vi "Get_Indexes_Connect_Dots&Min_ID-1.vi"(4 "(X,Y...) Tracks col":dbl[](array[numeric]), 5 "ID-dot col":u16[](array[numeric]), 6 "multiplier (x4)":i32, 7 "dot status":i16, 8 "initial ID":u16, 9 "Current Dot \nindex":i32, 10 "Dot coord":cluster{"X":dbl, "Y":dbl, "dX":dbl, "dY":dbl}, 11 "N elem. in col":i32) -> (0 "minimal ID \nbetween them":u16, 1 "amount":i32, 2 "Indexex Connec\ndots":i32[](array[numeric]))   [LabVIEW 2013]
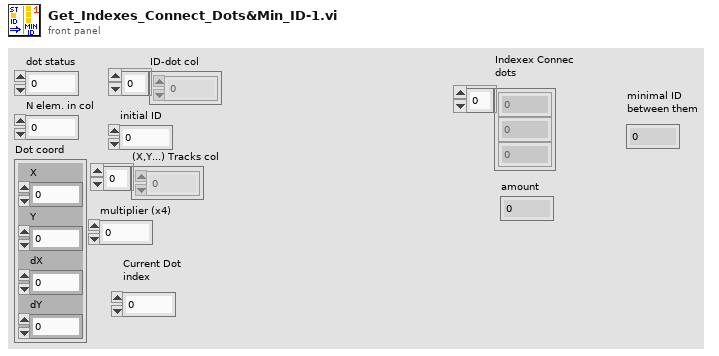
[diagram p1: front panel]
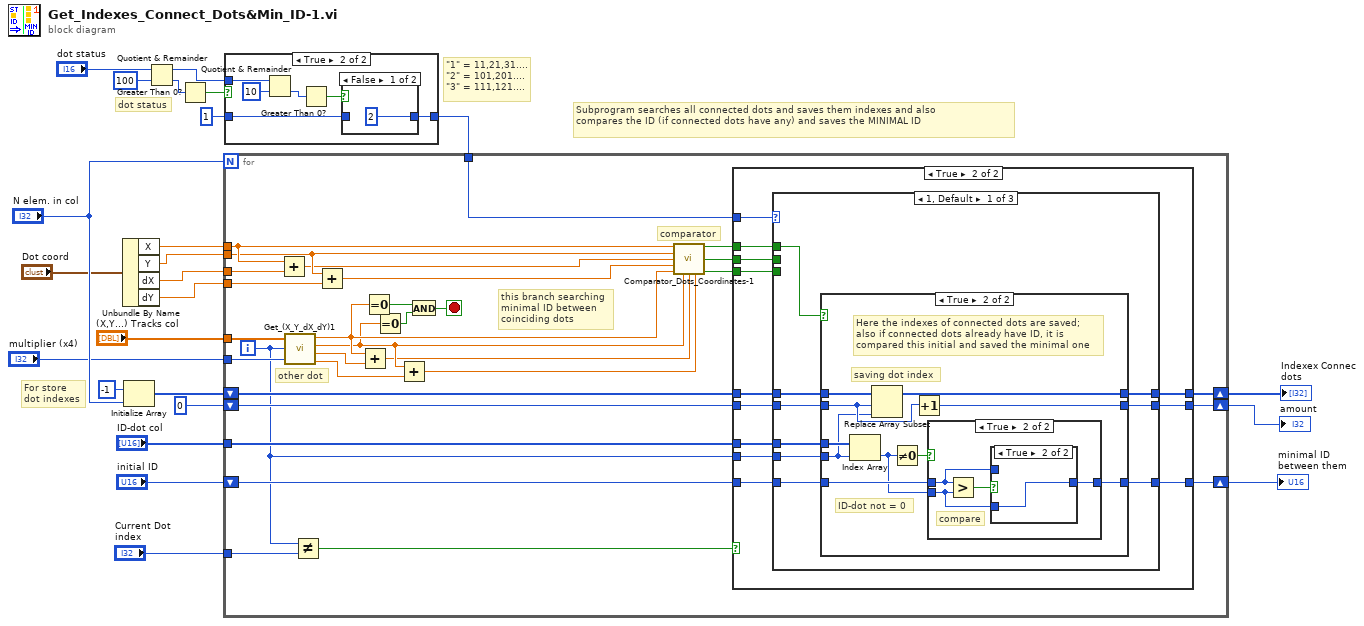
[diagram p0: block diagram]
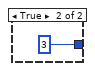
[diagram p3: hidden frame]
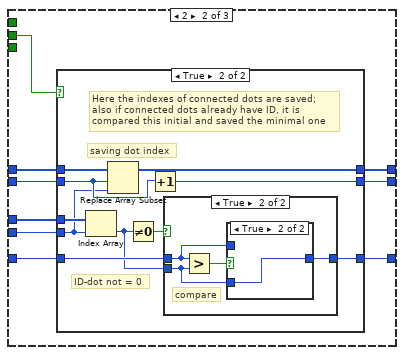
[diagram p8: hidden frame]
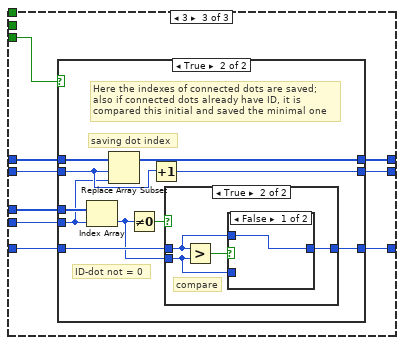
[diagram p12: hidden frame]
diagram:
  # "\"1\" = 11,21,31....\n\"2\" = 101,201....\n\"3\" = 111,121...."
  # "dot status"
  # "Subprogram searches all connected dots and saves them indexes and also\ncompares the ID (if connected dots have any) and saves the MINIMAL ID"
  # "For store \ndot indexes"
  n1 = Unbundle By Name("Dot coord") -> ("X"=w17:dbl, "Y"=w16:dbl, "dX"=w15:dbl, "dY"=w14:dbl)
  n2 = Initialize Array(-1 ("element"), "N elem. in col") -> (w23:i32[])
  n3 = Quotient & Remainder(x="dot status", y=i16 100) -> (x-y*floor(x/y)=w8:i16, floor(x/y)=w5:i16)
  n4 = Greater Than 0?(x=w5) -> (x > 0?=w6:bool)
  n5 = case shown="True" w6 {
    tunnel: 1 -> [w25 w27]
    tunnel: w8 -> [_ w31]
    tunnel: [w25 w26] -> w2
    frame False {
    }
    frame True {
      n6 = Quotient & Remainder(x=w31, y=i16 10) -> (floor(x/y)=w29:i16)  [unwired: 1 out]
      n7 = Greater Than 0?(x=w29) -> (x > 0?=w28:bool)
      n8 = case shown="False" w28 {
        tunnel: w27 -> [_ _]
        tunnel: [2 3] -> w26
        frame False {
        }
        frame True {
        }
      }
    }
  }
  n9 = for {
    N: "N elem. in col" -> [_]
    tunnel: "(X,Y...) Tracks col" -> [w64]
    tunnel: "multiplier (x4)" -> [w58]
    tunnel: w17 -> [w48]
    tunnel: w16 -> [w47]
    tunnel: w15 -> [w57]
    tunnel: w14 -> [w56]
    shift-right: [w53] -> w10
    shift-left: 0 -> [w54]
    shift-right: [w52] -> w11
    shift-left: w23 -> [w55]
    tunnel: "ID-dot col" -> [w51]
    shift-right: [w49] -> w9
    shift-left: "initial ID" -> [w50]
    tunnel: w2 -> [w37]
    tunnel: "Current Dot \nindex" -> [w35]
    i -> [w36]
    stop <- w61 stop-if-true
    # "comparator"
    # "this branch searching\nminimal ID between\ncoinciding dots"
    # "other dot"
    n10 = Add(x=w48, y=w57) -> (x+y=w46:dbl)
    n11 = call "Get_(X_Y_dX_dY)1.vi"("(X,Y,dX,dY)"=w64, "index"=w36, "multiplier"=w58) -> ("X"=w44:dbl, "Y"=w43:dbl, "dX"=w60:dbl, "dY"=w59:dbl)
    n12 = Not Equal?(x=w36, y=w35) -> (x != y?=w34:bool)
    n13 = Add(x=w47, y=w56) -> (x+y=w45:dbl)
    n14 = Add(x=w44, y=w60) -> (x+y=w42:dbl)
    n15 = Equal To 0?(x=w44) -> (x = 0?=w63:bool)
    n16 = Equal To 0?(x=w43) -> (x = 0?=w62:bool)
    n17 = Add(x=w43, y=w59) -> (x+y=w41:dbl)
    n18 = And(x=w63, y=w62) -> (x .and. y?=w61:bool)
    n19 = call "Comparator_Dots_Coordinates-1.vi"("X1"=w48, "Y1"=w47, "(X+dX)1"=w46, "(Y+dY)1"=w45, "X2"=w44, "Y2"=w43, "(X+dX)2"=w42, "(Y+dY)2"=w41) -> ("X1=X2,Y1=Y2 (1)"=w40:bool, "X1(2)=X2(2),Y1(2)=Y2(2) (2)"=w39:bool, "(1) OR (2) = (3)"=w38:bool)  [unwired: 5 in]
    n20 = case shown="True" w34 {
      tunnel: w55 -> [w67 w79]
      tunnel: w54 -> [w66 w78]
      tunnel: [w66 w77] -> w53
      tunnel: [w67 w76] -> w52
      tunnel: w51 -> [_ w75]
      tunnel: w36 -> [_ w74]
      tunnel: w50 -> [w65 w73]
      tunnel: [w65 w72] -> w49
      tunnel: w40 -> [_ w71]
      tunnel: w39 -> [_ w70]
      tunnel: w38 -> [_ w69]
      tunnel: w37 -> [_ w68]
      frame False {
      }
      frame True {
        n21 = case shown="1, Default" w68 {
          tunnel: w79 -> [w88 w117 w146]
          tunnel: w78 -> [w87 w116 w145]
          tunnel: [w81 w114 w139] -> w77
          tunnel: [w82 w115 w140] -> w76
          tunnel: w75 -> [w86 w113 w144]
          tunnel: w74 -> [w85 w112 w143]
          tunnel: w73 -> [w84 w111 w142]
          tunnel: [w80 w110 w138] -> w72
          tunnel: w69 -> [_ _ w141]
          tunnel: w70 -> [_ w109 _]
          tunnel: w71 -> [w83 _ _]
          frame 1, Default {
            n22 = case shown="True" w83 {
              tunnel: w88 -> [w91 w101]
              tunnel: w87 -> [w90 w98]
              tunnel: [w91 w100] -> w82
              tunnel: [w90 w99] -> w81
              tunnel: w86 -> [_ w97]
              tunnel: w85 -> [_ w95]
              tunnel: w84 -> [w89 w94]
              tunnel: [w89 w92] -> w80
              frame False {
              }
              frame True {
                # "ID-dot not = 0"
                # "Here the indexes of connected dots are saved;\nalso if connected dots already have ID, it is\ncompared this initial and saved the minimal one"
                # "saving dot index"
                n23 = Index Array(array=w97, index=w95) -> (element=w93:u16)
                n24 = Replace Array Subset(array=w101, new element=w95, index=w98) -> (w100:i32[])
                n25 = Not Equal To 0?(x=w93) -> (x != 0?=w96:bool)
                n26 = Increment(x=w98) -> (x+1=w99:i32)
                n27 = case shown="True" w96 {
                  tunnel: w94 -> [w102 w104]
                  tunnel: w93 -> [_ w105]
                  tunnel: [w102 w103] -> w92
                  frame False {
                  }
                  frame True {
                    # "compare"
                    n28 = Greater?(x=w104, y=w105) -> (0:w106:bool)
                    n29 = case shown="True" w106 {
                      tunnel: w105 -> [_ w108]
                      tunnel: [w107 w108] -> w103
                      tunnel: w104 -> [w107 _]
                      frame False {
                      }
                      frame True {
                      }
                    }
                  }
                }
              }
            }
          }
          frame 2 {
            n30 = case shown="True" w109 {
              tunnel: w117 -> [w120 w130]
              tunnel: w116 -> [w119 w127]
              tunnel: [w120 w129] -> w115
              tunnel: [w119 w128] -> w114
              tunnel: w113 -> [_ w126]
              tunnel: w112 -> [_ w124]
              tunnel: w111 -> [w118 w123]
              tunnel: [w118 w121] -> w110
              frame False {
              }
              frame True {
                # "ID-dot not = 0"
                # "Here the indexes of connected dots are saved;\nalso if connected dots already have ID, it is\ncompared this initial and saved the minimal one"
                # "saving dot index"
                n31 = Index Array(array=w126, index=w124) -> (element=w122:u16)
                n32 = Replace Array Subset(array=w130, new element=w124, index=w127) -> (w129:i32[])
                n33 = Not Equal To 0?(x=w122) -> (x != 0?=w125:bool)
                n34 = Increment(x=w127) -> (x+1=w128:i32)
                n35 = case shown="True" w125 {
                  tunnel: w123 -> [w131 w133]
                  tunnel: w122 -> [_ w134]
                  tunnel: [w131 w132] -> w121
                  frame False {
                  }
                  frame True {
                    # "compare"
                    n36 = Greater?(x=w133, y=w134) -> (0:w135:bool)
                    n37 = case shown="True" w135 {
                      tunnel: w134 -> [_ w137]
                      tunnel: [w136 w137] -> w132
                      tunnel: w133 -> [w136 _]
                      frame False {
                      }
                      frame True {
                      }
                    }
                  }
                }
              }
            }
          }
          frame 3 {
            n38 = case shown="True" w141 {
              tunnel: w146 -> [w149 w159]
              tunnel: w145 -> [w148 w156]
              tunnel: [w149 w158] -> w140
              tunnel: [w148 w157] -> w139
              tunnel: w144 -> [_ w155]
              tunnel: w143 -> [_ w153]
              tunnel: w142 -> [w147 w152]
              tunnel: [w147 w150] -> w138
              frame False {
              }
              frame True {
                # "ID-dot not = 0"
                # "Here the indexes of connected dots are saved;\nalso if connected dots already have ID, it is\ncompared this initial and saved the minimal one"
                # "saving dot index"
                n39 = Index Array(array=w155, index=w153) -> (element=w151:u16)
                n40 = Replace Array Subset(array=w159, new element=w153, index=w156) -> (w158:i32[])
                n41 = Not Equal To 0?(x=w151) -> (x != 0?=w154:bool)
                n42 = Increment(x=w156) -> (x+1=w157:i32)
                n43 = case shown="True" w154 {
                  tunnel: w152 -> [w160 w162]
                  tunnel: w151 -> [_ w163]
                  tunnel: [w160 w161] -> w150
                  frame False {
                  }
                  frame True {
                    # "compare"
                    n44 = Greater?(x=w162, y=w163) -> (0:w164:bool)
                    n45 = case shown="False" w164 {
                      tunnel: w163 -> [_ w166]
                      tunnel: [w165 w166] -> w161
                      tunnel: w162 -> [w165 _]
                      frame False {
                      }
                      frame True {
                      }
                    }
                  }
                }
              }
            }
          }
        }
      }
    }
  }
  "Indexex Connec\ndots" <- w11
  "amount" <- w10
  "minimal ID \nbetween them" <- w9
